vi "Get Object.vi"(8 "error in (no error)":errorcluster, 10 "Name Array":string[](array[string]), 11 "JSON Object in":refnum<class "JSON Value.lvclass">) -> (0 "error out":errorcluster, 1 "Sub-Item Names":string[](array[string]), 2 "Sub-Items":refnum<class "JSON Value.lvclass">[](array[class]), 3 "JSON Array out":refnum<class "JSON Value.lvclass">)   [LabVIEW 2020, in "Library Commun.lvlib" / "JSON Object.lvclass"]
uses:
  JSON Object.lvclass
  JSON Value/JSON Value.lvclass
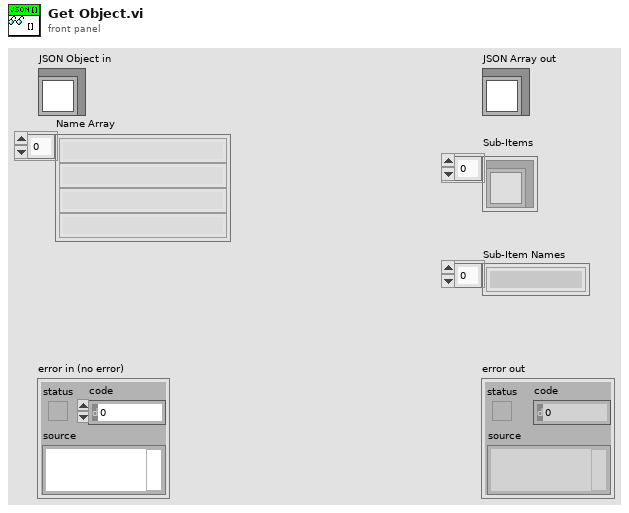
[diagram p1: front panel]
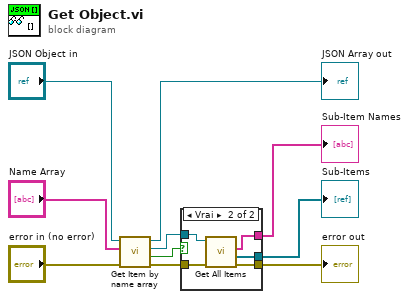
[diagram p0: block diagram]
diagram:
  n1 = call "Get Item by name array.vi"("error in (no error)"="error in (no error)", "Name Array"="Name Array", "JSON Value In"="JSON Object in") -> ("error out"=w10:errorcluster, "found"=w9:bool, "Value"=w8:refnum<class "JSON Value.lvclass">, "JSON Value Out"=→"JSON Array out":refnum<class "JSON Value.lvclass">)  [unwired: 5 in]
  n2 = case shown="Vrai" w9 {
    tunnel: w8 -> [_ w16]
    tunnel: [_ w13] -> w5
    tunnel: w10 -> [w11 w15]
    tunnel: [w11 w14] -> w4
    tunnel: [_ w12] -> w1
    frame False {
    }
    frame True {
      n3 = call-dynamic "Get All Items.vi"("error in (no error)"=w15, "JSON Value In"=w16) -> ("error out"=w14:errorcluster, "Values"=w13:refnum<class "JSON Value.lvclass">[], "Item Names"=w12:string[])  [unwired: 6 in, 1 out]
    }
  }
  "error out" <- w4
  "Sub-Items" <- w5
  "Sub-Item Names" <- w1
